vi "GetChannelFromNavX-MXPPin.vi"(10 "navX-MXP Pin Type":T1, 11 "navX-MXP Pin Number":u8) -> (3 "RoboRIO Channel Number":u8)   [LabVIEW 2014]
uses:
  navX-MXP_PinTypeDef.ctl
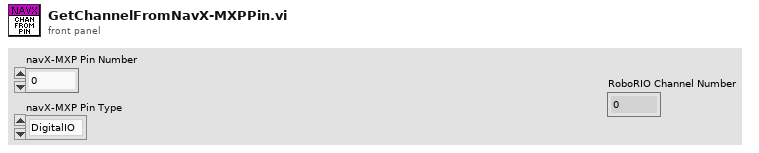
[diagram p1: front panel]
types:
  T1 = typedef "navX-MXP_PinTypeDef.ctl" = enum16{"DigitalIO", "PWM", "AnalogIn", "AnalogOut", ""}
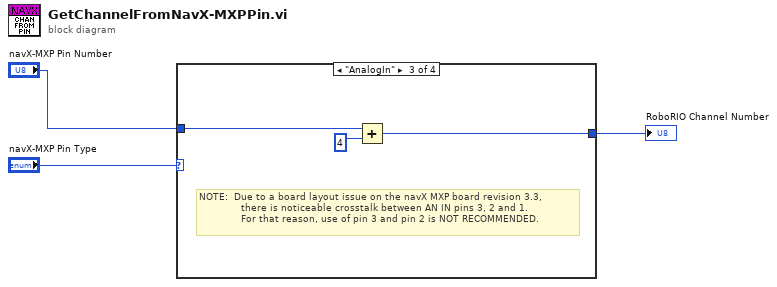
[diagram p0: block diagram]
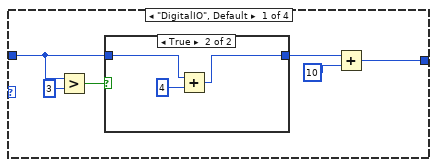
[diagram p2: hidden frame]
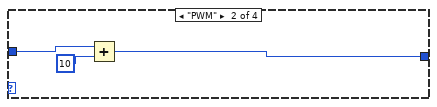
[diagram p4: hidden frame]
diagram:
  n1 = case shown="\"AnalogIn\"" "navX-MXP Pin Type" {
    tunnel: "navX-MXP Pin Number" -> [w6 w15 w18 w20]
    tunnel: [w4 w14 w17 w20] -> w2
    frame "DigitalIO", Default {
      n2 = Greater?(x=w6, y=3) -> (0:w7:bool)
      n3 = case shown="True" w7 {
        tunnel: w6 -> [w10 w12]
        tunnel: [w10 w11] -> w5
        frame False {
        }
        frame True {
          n4 = Add(x=w12, y=4) -> (x+y=w11:i32)
        }
      }
      n5 = Add(x=w5, y=10) -> (x+y=w4:i32)
    }
    frame "PWM" {
      n6 = Add(x=w15, y=10) -> (x+y=w14:i32)
    }
    frame "AnalogIn" {
      # "NOTE:  Due to a board layout issue on the navX MXP board revision 3.3, \n              there is noticeable crosstalk between AN IN pins 3, 2 and 1.\n              For that reason, use of pin 3 and pin 2 is NOT RECOMMENDED."
      n7 = Add(x=w18, y=4) -> (x+y=w17:i32)
    }
    frame "AnalogOut" {
    }
  }
  "RoboRIO Channel Number" <- w2
